vi "Byte Array to Supported Schemes.vi"(1 "Buffer":u8[](array[numeric])) -> (0 "Supported Schemes":T1[](array[typedef]))   [LabVIEW 2018, in "Toolkit.lvlib" / "Session.lvclass"]
doc: "Converts a byte array of comma-delimited string values into a list of supported authentication schemes by the remote SSH/SFTP server."
uses:
  Session.lvclass
  Type Definitions/User Authentication Schemes.ctl
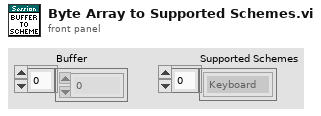
[diagram p1: front panel]
types:
  T1 = typedef "Toolkit.lvlib/Session.lvclass/User Authentication Schemes.ctl" = enum16{"Keyboard", "Password", "Public Key"}
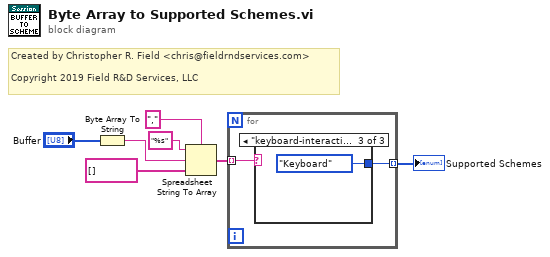
[diagram p0: block diagram]
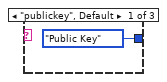
[diagram p2: hidden frame]
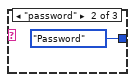
[diagram p3: hidden frame]
diagram:
  # "Created by Christopher R. Field <chris@fieldrndservices.com>\n\nCopyright 2019 Field R&D Services, LLC"
  n1 = Byte Array To String(unsigned byte array="Buffer") -> (string=w1:string)
  n2 = Spreadsheet String To Array(delimiter (Tab)=",", format string="%s", spreadsheet string=w1, array type (2D Dbl)=string[] []) -> (array=w5:string[])
  n3 = for {
    tunnel: w5 -> [w9] mode=indexing
    tunnel: [w8] -> w7 mode=indexing
    n4 = case shown="\"keyboard-interactive\"" w9 {
      tunnel: [User_Authentication_Schemes."Public Key" ("Scheme") User_Authentication_Schemes."Password" ("Scheme") User_Authentication_Schemes."Keyboard" ("Scheme")] -> w8
      frame "publickey", Default {
      }
      frame "password" {
      }
      frame "keyboard-interactive" {
      }
    }
  }
  "Supported Schemes" <- w7
